vi "Reverse saturation current.vi"(6 "T":dbl, 9 "N_s":dbl, 10 "V_OC":dbl, 11 "I_sc":dbl) -> (3 "I_rs":dbl)   [LabVIEW 2024]
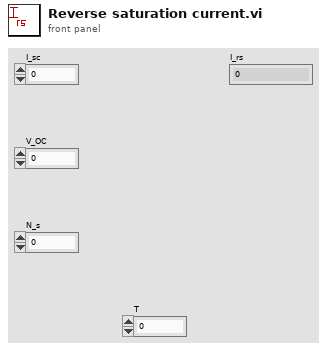
[diagram p1: front panel]
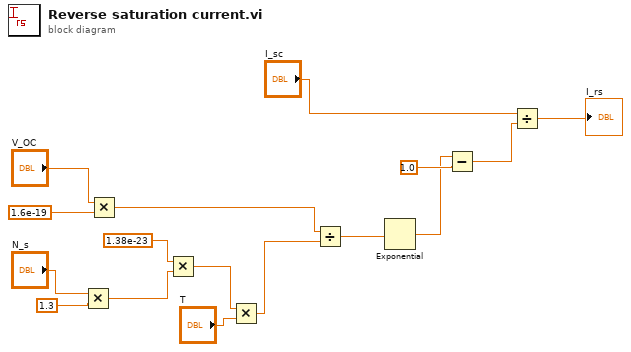
[diagram p0: block diagram]
diagram:
  n1 = Multiply(x="N_s", y=1.3) -> (x*y=w5:dbl)
  n2 = Multiply(x="V_OC", y=1.6e-19) -> (x*y=w9:dbl)
  n3 = Multiply(x=1.38e-23, y=w5) -> (x*y=w7:dbl)
  n4 = Multiply(x=w7, y="T") -> (x*y=w10:dbl)
  n5 = Divide(x=w9, y=w10) -> (x/y=w11:dbl)
  n6 = Exponential(1:w11) -> (0:w12:dbl)
  n7 = Subtract(x=w12, y=1.0) -> (x-y=w15:dbl)
  n8 = Divide(x="I_sc", y=w15) -> (x/y=→"I_rs":dbl)
